vi "Save_TDMS_file.vi"(6 "ADC_data":u16[][](array[numeric]), 10 "File Path":string, 11 "Save Results":bool) -> ()   [LabVIEW 2017]
uses:
  Measurement_Param_Global_Var.vi
  Board_Global_Var.vi
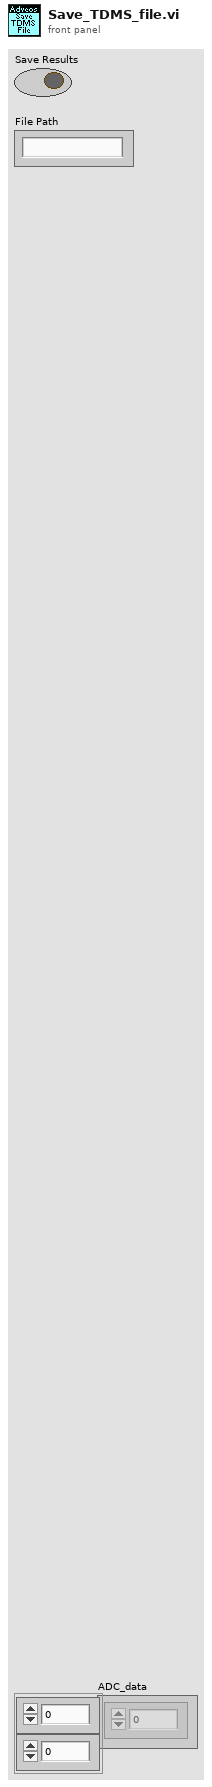
[diagram p1: front panel]
types:
  T1 = cluster{"Cap Trim 1 ADC1":u16, "Cap Trim 2 ADC1":u16, "Cap Trim 1 ADC2":u16, "Cap Trim 2 ADC2":u16, "Pipestage Bias Current (36:0)":u64, "ADC Bias Current (5:0)":u8, "ADC2 En":bool, "ADC1 En":bool, "Bias Cur En":bool, "ADC Bias En":bool, "Bias from\nBGR":bool, "Bias Cur\nSelector":bool, "ADC Bias\nSelector":bool, "BGR \nPD":bool, "Bypass\nBGR":bool, "Start-up BGR\nPwr-up 1":bool, "Start-up BGR\nPwr-up 2":bool, "Current Test MUX":u8, "Int Vref":bool, "Int Vref 2":bool, "S/H  En":bool, "Vcm Sel":bool, "Vcm Sel 2":bool, "ADC Data Out":u8, "ADC1 Clk En":bool, "ADC2 Clk En":bool, "ADC \nPads En":bool}
  T2 = cluster{"Sweep Selection":enum32{"Cap Trim", "Bias Current", "Vreference"}, "Cap Trim 1 ADC1":u16, "Step size Cap Neg":u16, "Nb of steps Cap Neg":u16, "Cap_Trim_Neg En":bool, "Cap Trim Pos":u16, "Step size Cap Pos":u16, "Nb of steps Cap Pos":u16, "Cap_Trim_Pos En":bool, "PipeStage Bias":u64, "Step size PipeStage":u16, "Nb of steps PipeStage":u64, "PipeStage Bias En":bool, "ADC Bias":u8, "Step size ADC Bias":u16, "Nb of steps ADC Bias":u8, "ADC Bias En":bool}
  T3 = enum16{"open", "open or create", "create or replace", "create", "open (read-only)"}
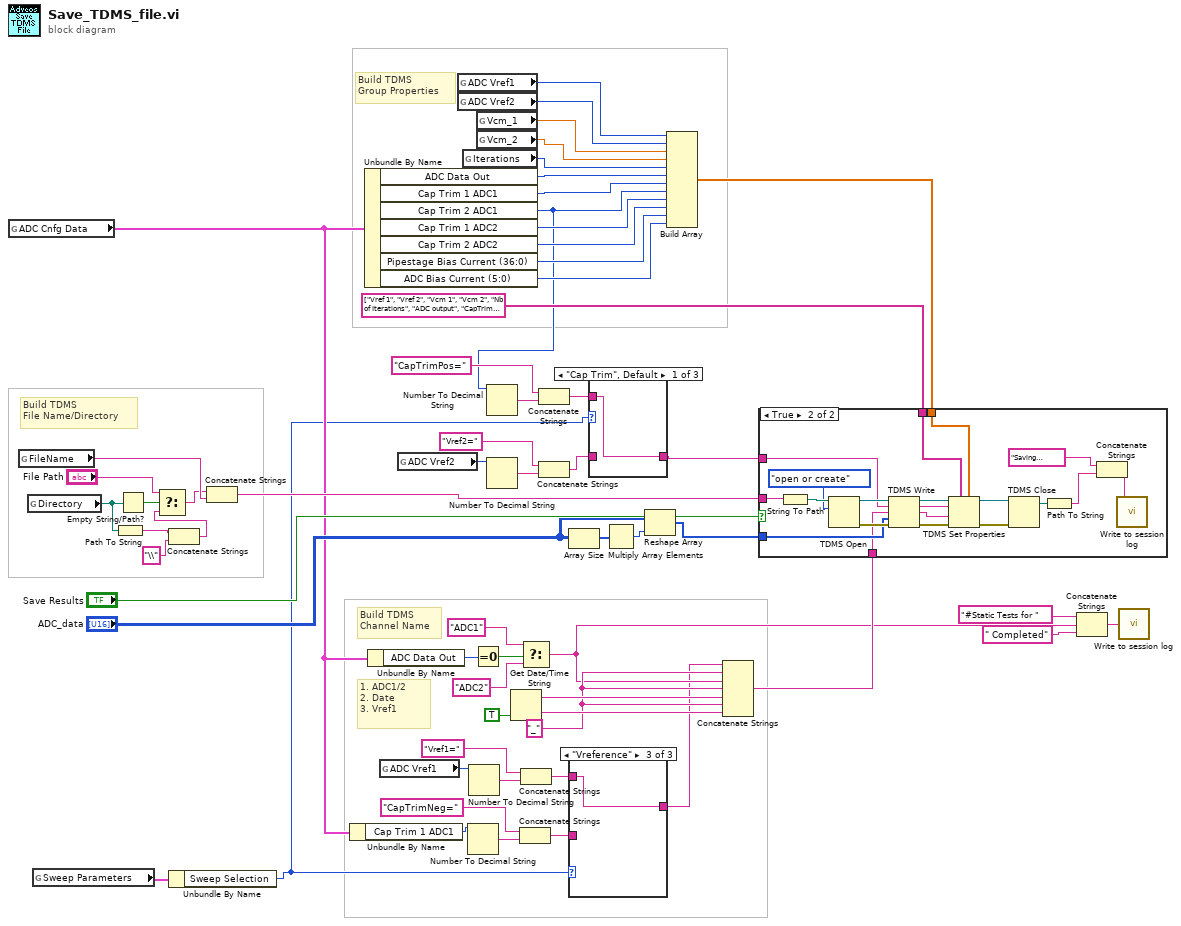
[diagram p0: block diagram]
diagram:
  w24 = "_" ("string")
  # "Build TDMS \nFile Name/Directory"
  # "Build TDMS \nGroup Properties"
  # "1. ADC1/2\n2. Date\n3. Vref1"
  # "Build TDMS \nChannel Name"
  n1 = global read "Measurement_Param_Global_Var.vi" "ADC Cnfg Data"() -> (w12:T1)
  n2 = global read "Board_Global_Var.vi" "FileName"() -> (w50:string)
  n3 = global read "Board_Global_Var.vi" "Directory"() -> (w33:path)
  n4 = global read "Measurement_Param_Global_Var.vi" "Sweep Parameters"() -> (w16:T2)
  n5 = Path To String(path=w33) -> (string=w26:string)
  n6 = Empty String/Path?(string/path=w33) -> (empty?=w35:bool)
  n7 = Concatenate Strings(w26, "\\" ("string")) -> (w25:string)
  n8 = Select(t="File Path", s=w35, f=w25) -> (s? t:f=w32:string)
  n9 = Unbundle By Name(w16) -> ("Sweep Selection"=w4:enum32{"Cap Trim", "Bias Current", "Vreference"})
  n10 = Concatenate Strings(w32, w50) -> (w51:string)
  n11 = Unbundle By Name(w12) -> ("Cap Trim 1 ADC1"=w11:u16)
  n12 = Unbundle By Name(w12) -> ("ADC Data Out"=w42:u8, "Cap Trim 1 ADC1"=w43:u16, "Cap Trim 2 ADC1"=w5:u16, "Cap Trim 1 ADC2"=w44:u16, "Cap Trim 2 ADC2"=w45:u16, "Pipestage Bias Current (36:0)"=w46:u64, "ADC Bias Current (5:0)"=w47:u8)
  n13 = Unbundle By Name(w12) -> ("ADC Data Out"=w56:u8)
  n14 = global read "Measurement_Param_Global_Var.vi" "ADC Vref1"() -> (w30:u16)
  n15 = global read "Measurement_Param_Global_Var.vi" "ADC Vref2"() -> (w18:u16)
  n16 = global read "Measurement_Param_Global_Var.vi" "ADC Vref1"() -> (w37:u16)
  n17 = global read "Measurement_Param_Global_Var.vi" "ADC Vref2"() -> (w38:u16)
  n18 = global read "Measurement_Param_Global_Var.vi" "Iterations"() -> (w41:u16)
  n19 = Number To Decimal String(number=w11) -> (decimal integer string=w14:string)  [unwired: 1 in]
  n20 = Number To Decimal String(number=w30) -> (decimal integer string=w29:string)  [unwired: 1 in]
  n21 = Equal To 0?(x=w56) -> (x = 0?=w57:bool)
  n22 = global read "Measurement_Param_Global_Var.vi" "Vcm_1"() -> (w39:dbl)
  n23 = global read "Measurement_Param_Global_Var.vi" "Vcm_2"() -> (w40:dbl)
  n24 = Number To Decimal String(number=w5) -> (decimal integer string=w6:string)  [unwired: 1 in]
  n25 = Number To Decimal String(number=w18) -> (decimal integer string=w19:string)  [unwired: 1 in]
  n26 = Get Date/Time String(want seconds? (F)=TRUE) -> (date string=w60:string, time string=w61:string)  [unwired: 2 in]
  n27 = Concatenate Strings("CapTrimNeg=" ("t"), w14) -> (w9:string)
  n28 = Select(t="ADC1", s=w57, f="ADC2") -> (s? t:f=w15:string)
  n29 = Concatenate Strings("Vref1=" ("t"), w29) -> (w10:string)
  n30 = Concatenate Strings("CapTrimPos=" ("t"), w6) -> (w3:string)
  n31 = Concatenate Strings("Vref2=" ("t"), w19) -> (w2:string)
  n32 = Array Size(array="ADC_data") -> (size(s)=w23:i32[])
  n33 = case shown="\"Vreference\"" w4 {
    tunnel: w10 -> [_ _ w63]
    tunnel: w9 -> [w62 _ _]
    tunnel: [w62 _ w63] -> w8
    frame "Cap Trim", Default {
    }
    frame "Bias Current" {
    }
    frame "Vreference" {
    }
  }
  n34 = case shown="\"Cap Trim\", Default" w4 {
    tunnel: w3 -> [w64 _ _]
    tunnel: w2 -> [_ _ w65]
    tunnel: [w64 _ w65] -> w1
    frame "Cap Trim", Default {
    }
    frame "Bias Current" {
    }
    frame "Vreference" {
    }
  }
  n35 = Multiply Array Elements(1:w23) -> (0:w22:i32)
  n36 = Reshape Array("ADC_data", w22) -> (w20:u16[])
  n37 = Build Array(w37, w38, w39, w40, w41, w42, w43, w5, w44, w45, w46, w47) -> (w36:dbl[])
  n38 = Concatenate Strings(w8, w24, w15, w24, w60, w24, w61) -> (w28:string)
  n39 = case shown="True" "Save Results" {
    tunnel: w28 -> [_ w68]
    tunnel: w51 -> [_ w81]
    tunnel: string[] ["Vref 1", "Vref 2", "Vcm 1", "Vcm 2", "Nb of Iterations", "ADC output", "CapTrim1 ADC1", "CapTrim2 ADC1", "CapTrim1 ADC2", "CapTrim2 ADC2", "Pipe Stage Current", "ADC Bias Current"] -> [_ w72]
    tunnel: w36 -> [_ w71]
    tunnel: w20 -> [_ w69]
    tunnel: w1 -> [_ w66]
    frame False {
    }
    frame True {
      n40 = String To Path(string=w81) -> (path=w85:path)
      n41 = TDMS Open(10:T3."open or create" ("operation (0:open)"), 11:w85) -> (0:w82:errorcluster, 3:w83:refnum<k34>)  [unwired: 5 in]
      n42 = TDMS Write(0:w83, 5:w66, 7:w68, 9:w69, 11:w82) -> (4:w73:refnum<k34>, 6:w70:string, 8:w67:string, 15:w76:errorcluster)  [unwired: 1 in]
      n43 = TDMS Set Properties(5:w71, 7:w72, 8:w76, 9:w67, 10:w70, 11:w73) -> (0:w75:errorcluster, 3:w74:refnum<k34>)  [unwired: 2 out]
      n44 = TDMS Close(8:w75, 11:w74) -> (3:w80:path)  [unwired: 1 out]
      n45 = Path To String(path=w80) -> (string=w77:string)
      n46 = Concatenate Strings("Saving Results to file " ("string"), w77) -> (w79:string)
      n47 = call "Write to session log.vi"("Session string"=w79) -> ()  [unwired: 1 in]
    }
  }
  n48 = Concatenate Strings("#Static Tests for " ("Session string"), w15, " Completed" ("string")) -> (w52:string)
  n49 = call "Write to session log.vi"("Session string"=w52) -> ()  [unwired: 1 in]
